vi "preBuildLUT.vi"() -> ()   [LabVIEW 2021]
uses:
  <vilib>/Analysis/1siggen.llb/Ramp Pattern by Samples.vi
  <vilib>/Analysis/NI_AALBase.lvlib
panel:
  out "colours":u32[](array[colorbox])
  out "values":dbl[](array[numeric])
  out "colour":u32(colorbox)
  in  "value":dbl
  in  "samples":i32=128
  in  "rampMarkers":cluster{"value":dbl, "colour":u32}[](array[cluster])
  out "ramper":dbl(ramp)
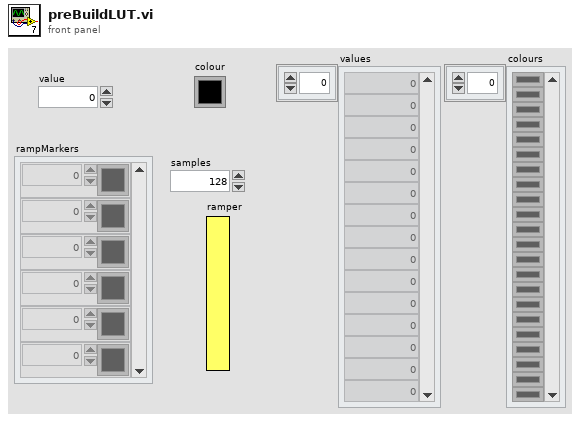
[diagram p1: front panel]
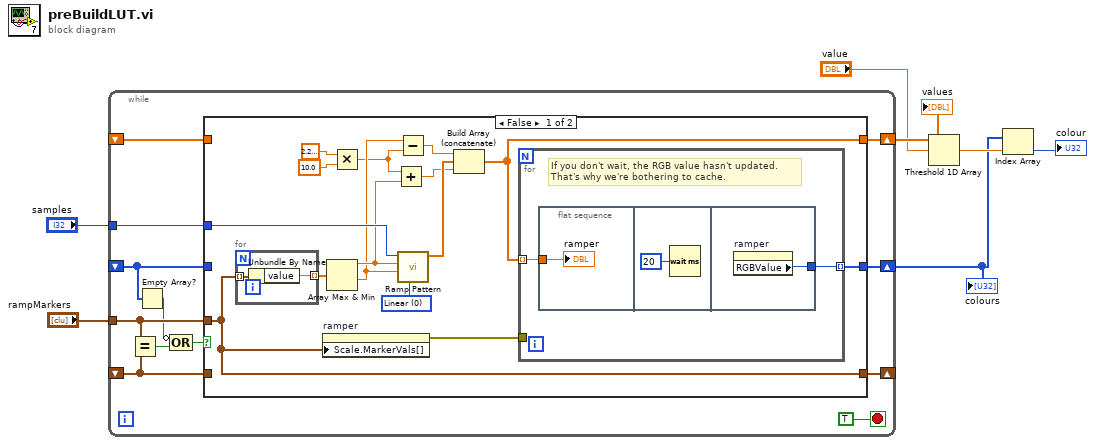
[diagram p0: block diagram]
diagram:
  n1 = while {
    tunnel: "rampMarkers" -> [w13]
    shift-right: [w19] -> w7
    shift-left: _ -> [w16]
    shift-right: [w18] -> w5
    shift-left: _ -> [w9]
    shift-right: [w15] -> _
    shift-left: _ -> [w12]
    tunnel: "samples" -> [w8]
    stop <- TRUE stop-if-true
    n2 = Equal?(x=w13, y=w12) -> (x = y?=w14:bool)
    n3 = Empty Array?(array=w9) -> (empty?=w10:bool)
    n4 = Compound Arithmetic op=OR(invert w10, w14) -> (w11:bool)
    n5 = case shown="False" w11 {
      tunnel: [w24 w44] -> w19
      tunnel: [w31 w43] -> w18
      tunnel: w13 -> [w29 _]
      tunnel: w16 -> [_ w44]
      tunnel: w9 -> [_ w43]
      tunnel: [w29 w42] -> w15
      tunnel: w12 -> [_ w42]
      tunnel: w8 -> [w28 _]
      frame False {
        w34 = u16 0 items=["Linear", "Logarithmic"] ("type")
        n6 = for {
          tunnel: w29 -> [w36] mode=indexing
          tunnel: [w35] -> w30 mode=indexing
          n7 = Unbundle By Name(w36) -> ("value"=w35:dbl)
        }
        n8 = property on="ramper" class="ColRmp (strict)"("Scale.MarkerVals[]"=w29) -> (error out=w33:errorcluster)  [unwired: 2 in, 1 out]
        n9 = Array Max & Min(array=w30) -> (max value=w26:dbl, min value=w25:dbl)  [unwired: 2 out]
        n10 = Multiply(x=2.220446049250313e-16, y=10.0) -> (x*y=w21:dbl)
        n11 = Add(x=w21, y=w26) -> (x+y=w22:dbl)
        n12 = Subtract(x=w25, y=w21) -> (x-y=w23:dbl)
        n13 = call-poly <vilib>:"Ramp Pattern.vi"("type"=w34, "start"=w25, "end"=w26, "samples"=w28) -> ("Ramp Pattern"=w32:dbl[])  [unwired: 6 in, 1 out]
        n14 = Build Array (concatenate)(w23, w32, w22) -> (w24:dbl[])
        n15 = for {
          tunnel: w24 -> [w38] mode=indexing
          tunnel: w33 -> [_]
          tunnel: [w37] -> w31 mode=indexing
          # "If you don't wait, the RGB value hasn't updated.\nThat's why we're bothering to cache."
          n16 = flat-sequence {
            tunnel: w38 -> [w39]
            tunnel: [w41] -> w37
            frame #0 {
              "ramper" <- w39
            }
            frame #1 {
              n17 = Wait (ms)(milliseconds to wait=u32 20) -> ()  [unwired: 1 out]
            }
            frame #2 {
              n18 = property on="ramper" class="ColRmp (strict)"() -> ("RGBValue"=w41:u32)  [unwired: 2 in, 2 out]
            }
          }
        }
      }
      frame True {
      }
    }
  }
  "values" <- w7
  "colours" <- w5
  n19 = Threshold 1D Array(2:"value", 3:w7) -> (0:w6:dbl)  [unwired: 1 in]
  n20 = Index Array(array=w5, index=w6) -> (element=→"colour":u32)
